vi "mandar_email.vi"() -> ()   [LabVIEW 2019]
panel:
  out "error out":errorcluster
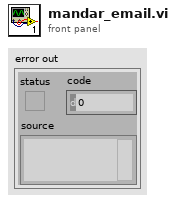
[diagram p1: front panel]
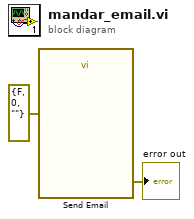
[diagram p0: block diagram]
diagram:
  n1 = call "Send Email"("error in"=errorcluster {"status"=FALSE, "code"=0, "source"=""}) -> ("error out"=→"error out":errorcluster)  [unwired: 10 in]
